vi "Calculate Delay and Wait.vi"(5 "wait limits (s)":cluster{"minimum":dbl, "maximum":dbl}={"minimum"=0.0, "maximum"=10.0}, 8 "expected interval (s)":dbl, 9 "previous time stamp":timestamp) -> (3 "new time stamp":timestamp)   [LabVIEW 2024, in "DSA_CFG_ACQ.lvlib"]
uses:
  DSA_CFG_ACQ.lvlib
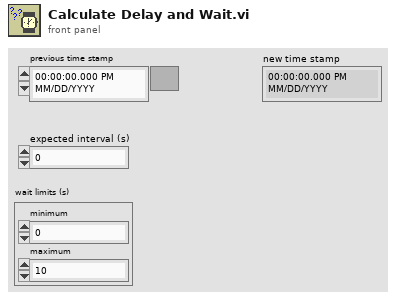
[diagram p1: front panel]
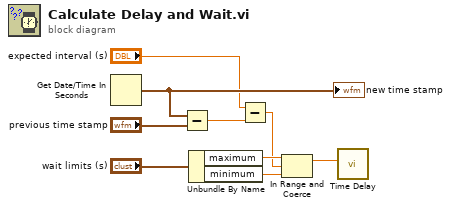
[diagram p0: block diagram]
diagram:
  n1 = Get Date/Time In Seconds() -> (seconds since 1Jan1904=w8:timestamp)
  "new time stamp" <- w8
  n2 = Subtract(x=w8, y="previous time stamp") -> (x-y=w3:dbl)
  n3 = Unbundle By Name("wait limits (s)") -> ("maximum"=w6:dbl, "minimum"=w5:dbl)
  n4 = Subtract(x="expected interval (s)", y=w3) -> (x-y=w4:dbl)
  n5 = In Range and Coerce(upper limit=w6, x=w4, lower limit=w5) -> (coerced(x)=w1:dbl)  [unwired: 1 out]
  n6 = call "Time Delay"("Delay Time (s)"=w1) -> ()  [unwired: 10 in, 1 out]
